vi "Channel 0 Individual Tube check (Reperpouse for Brute Force).vi"(5 "Individual Tube Current In":dbl[](array[numeric]), 6 "error in (no error)":errorcluster, 7 "Failed Tubes In":string[](array[string]), 8 "BoardHandle in":T1, 9 "Barcodes in":string[](array[string]), 10 "Tube #":i32, 11 "Channel # in":i32) -> (0 "BoardHandle out":T1, 1 "error out":errorcluster, 2 "Failed Tubes":string[](array[string]), 3 "Actual Voltage Level (V) 2":dbl format="%#_13g", 4 "Individual Tube Current (Nano Amps)":dbl[](array[numeric]))   [LabVIEW 2020]
uses:
  SUB VI Dark Current Test Files 2018 For Drop Box/Program Files (x86)/National Instruments/LabVIEW 2020/instr.lib/CAEN PSM/CAEN PSM.lvlib
panel:
  out "Recorded Current\nfor Previous Tube":dbl format="%#_13g"
  out "Next Measurment":string
  # "future developement"
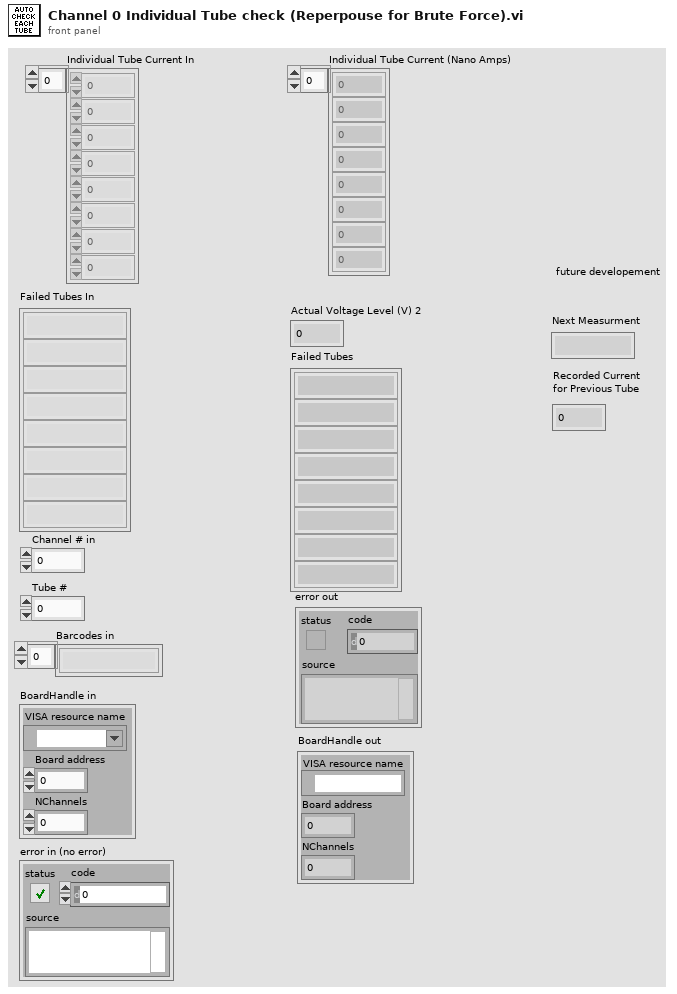
[diagram p1: front panel]
types:
  T1 = cluster{"VISA resource name":refnum<visa-resource-name>, "Board address":u8, "NChannels":u8}
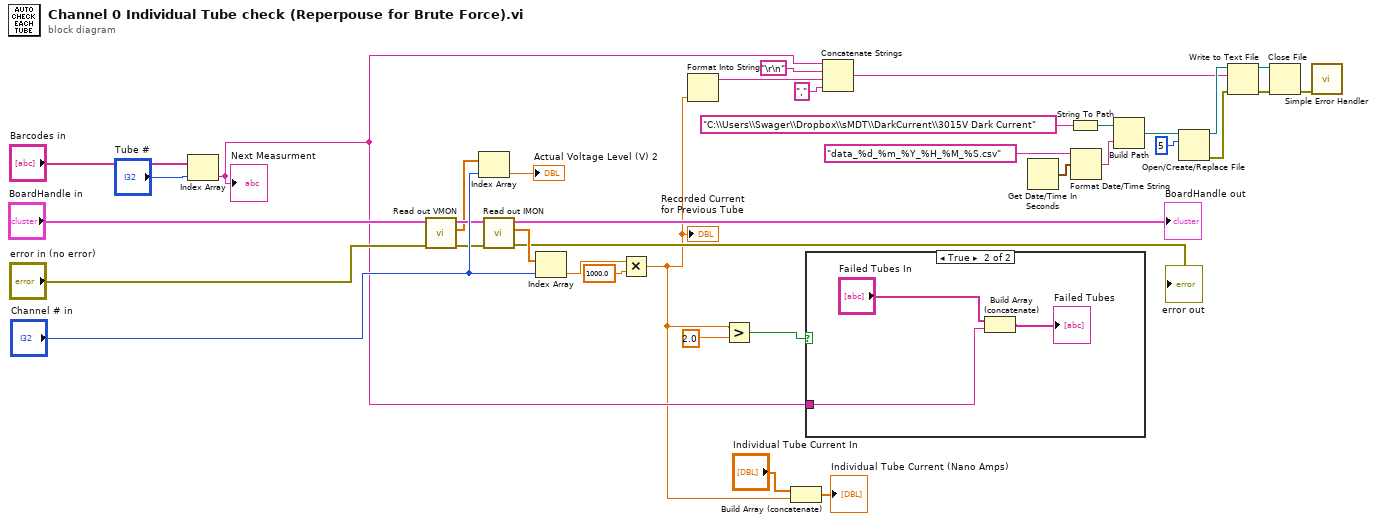
[diagram p0: block diagram]
diagram:
  n1 = Index Array(array="Barcodes in", index="Tube #") -> (element=w4:string)
  "Next Measurment" <- w4
  n2 = call "Read out VMON.vi"("error in (no error)"="error in (no error)", "BoardHandle"="BoardHandle in") -> ("error out"=w10:errorcluster, "VMon values (V)"=w8:dbl[], "BoardHandle out"=w9:T1)  [unwired: 7 in]
  n3 = Index Array(array=w8, index="Channel # in") -> (element=→"Actual Voltage Level (V) 2":dbl)
  n4 = call "Read out IMON.vi"("error in (no error)"=w10, "BoardHandle"=w9) -> ("error out"=→"error out":errorcluster, "IMon values (uA)"=w13:dbl[], "BoardHandle out"=→"BoardHandle out":T1)  [unwired: 6 in, 1 out]
  n5 = Index Array(array=w13, index="Channel # in") -> (element=w11:dbl)
  n6 = Multiply(x=w11, y=1000.0) -> (x*y=w3:dbl)
  "Recorded Current\nfor Previous Tube" <- w3
  n7 = Format Into String(w3) -> (resulting string=w14:string)  [unwired: 3 in, 1 out]
  n8 = Greater?(x=w3, y=2.0) -> (0:w31:bool)
  n9 = Build Array (concatenate)("Individual Tube Current In", w3) -> (→"Individual Tube Current (Nano Amps)":dbl[])
  n10 = case shown="True" w31 {
    tunnel: w4 -> [_ w38]
    frame False {
    }
    frame True {
      n11 = Build Array (concatenate)("Failed Tubes In", w38) -> (→"Failed Tubes":string[])
    }
  }
  n12 = Concatenate Strings(w4, "\r\n", w14, ",") -> (w17:string)
  n13 = Get Date/Time In Seconds() -> (seconds since 1Jan1904=w27:timestamp)
  n14 = String To Path(string="C:\\Users\\Swager\\Dropbox\\sMDT\\DarkCurrent\\3015V Dark Current") -> (path=w26:path)
  n15 = Format Date/Time String(time format string (%c)="data_%d_%m_%Y_%H_%M_%S.csv", seconds (now)=w27) -> (date/time string=w28:string)  [unwired: 1 in]
  n16 = Build Path(base path=w26, name or relative path=w28) -> (appended path=w24:path)
  n17 = Open/Create/Replace File(file path (use dialog)=w24, operation (0:open)=5) -> (refnum out=w23:refnum<file>, error out=w22:errorcluster)  [unwired: 4 in, 1 out]
  n18 = Write to Text File(file (use dialog)=w23, text=w17, error in=w22) -> (refnum out=w21:refnum<file>, error out=w20:errorcluster)  [unwired: 1 in, 1 out]
  n19 = Close File(refnum=w21, error in=w20) -> (error out=w19:errorcluster)  [unwired: 1 out]
  n20 = call <vilib>:"Simple Error Handler.vi"("error in (no error)"=w19) -> ()  [unwired: 4 in, 5 out]
